vi "Access Levels.vi"(4 "Setup Menu Passwords":T1={"Level 1 Password"="123", "Level 2 Password"="228", "Level 3 Password"="3228679"}, 5 "Action":enum8{"Set Codes", "Get Level"}(ring)=enum."Get Level") -> (2 "Level":u8)   [LabVIEW 2013]
doc: "Functional global that allows the pass codes to be set or checked. When we are checking the existing pass codes against user entered ones, we will call the numeric key pad to allow the user to enter the new code."
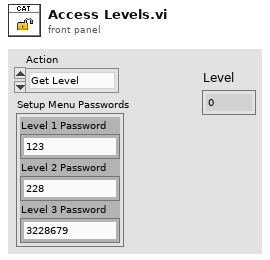
[diagram p1: front panel]
types:
  T1 = cluster{"Level 1 Password":string, "Level 2 Password":string, "Level 3 Password":string}
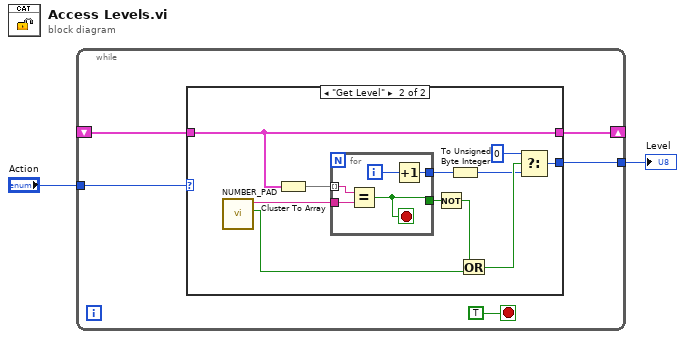
[diagram p0: block diagram]
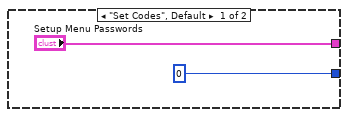
[diagram p2: hidden frame]
diagram:
  n1 = while {
    tunnel: [w7] -> w2
    tunnel: "Action" -> [w6]
    shift-right: [w5] -> _
    shift-left: _ -> [w4]
    stop <- TRUE stop-if-true
    n2 = case shown="\"Get Level\"" w6 {
      tunnel: [u8 0 ("t") w12] -> w7
      tunnel: ["Setup Menu Passwords" w20] -> w5
      tunnel: w4 -> [_ w20]
      frame "Set Codes", Default {
      }
      frame "Get Level" {
        n3 = call "NUMBER_PAD.vi"() -> ("Cancel?"=w15:bool, "number (out)"=w18:string)  [unwired: 10 in]
        n4 = Cluster To Array(cluster=w20) -> (array=w19:string[])
        n5 = for {
          tunnel: w19 -> [w25] mode=indexing
          tunnel: w18 -> [w24]
          tunnel: [w22] -> w11
          tunnel: [w21] -> w17
          i -> [w23]
          stop <- w21 stop-if-true
          n6 = Equal?(x=w25, y=w24) -> (x = y?=w21:bool)
          n7 = Increment(x=w23) -> (x+1=w22:i32)
        }
        n8 = Not(x=w17) -> (.not. x?=w16:bool)
        n9 = To Unsigned Byte Integer(number=w11) -> (unsigned 8bit integer=w10:u8)
        n10 = Or(x=w16, y=w15) -> (x .or. y?=w14:bool)
        n11 = Select(t=u8 0, s=w14, f=w10) -> (s? t:f=w12:u8)
      }
    }
  }
  "Level" <- w2
